vi "Display Results.vi"(8 "error in (no error)":errorcluster, 11 "Results in":refnum<class "Results.lvclass">) -> (0 "error out":errorcluster, 3 "Results out":refnum<class "Results.lvclass">)   [LabVIEW 2016, in "Result Actor.lvlib" / "Results.lvclass"]
uses:
  <userlib>/Common Components/Results/Results.lvclass
  <userlib>/Common Components/Results/Results.lvclass/Results.ctl
  <userlib>/Common Components/Results/Read Device Names Used.vi
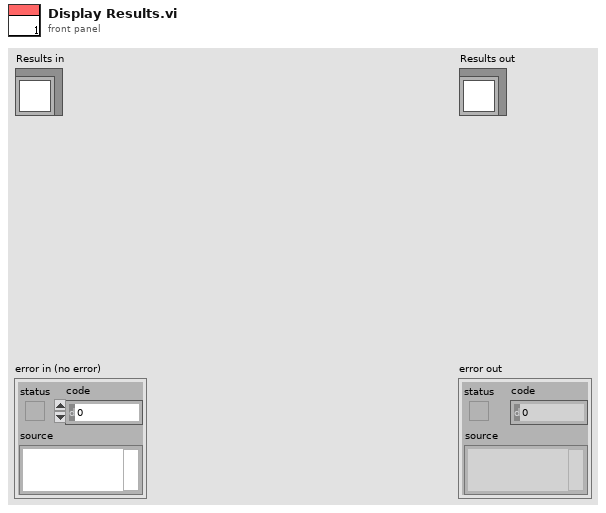
[diagram p1: front panel]
types:
  T1 = typedef "Result Actor.lvlib/Results.lvclass/UI References.ctl" = cluster{"Stop Button":refnum<vi>, "Waveform Graph":refnum<vi>, "Result Name":refnum<vi>, "Pass?":refnum<vi>}
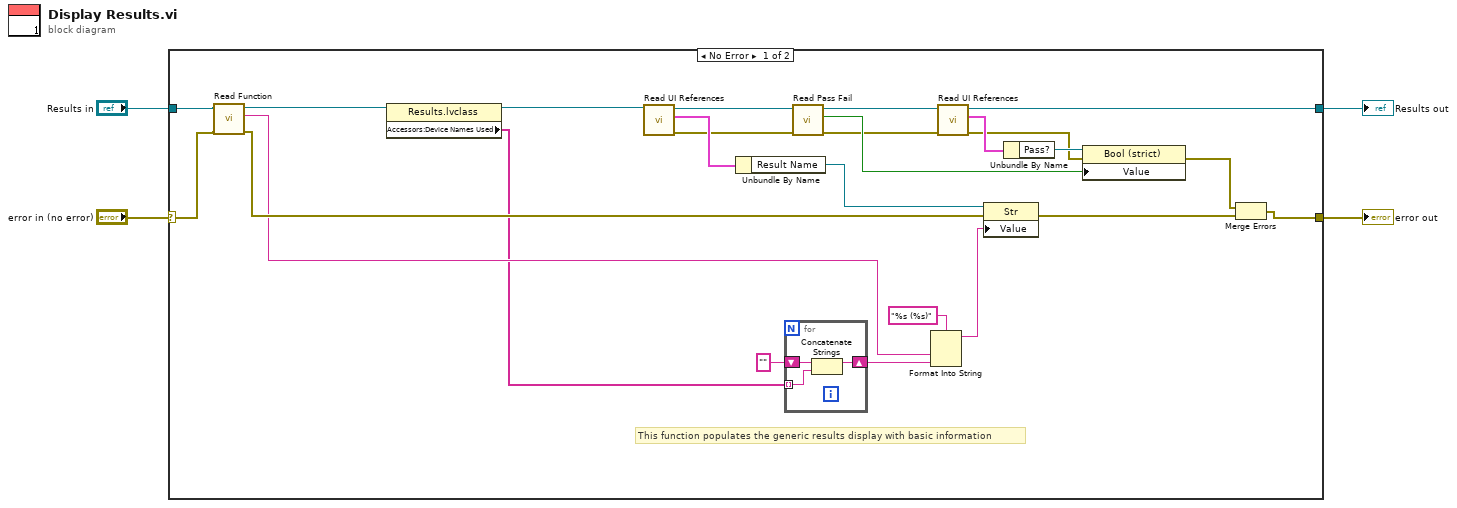
[diagram p0: block diagram]
diagram:
  n1 = case shown="No Error" "error in (no error)" {
    selector: "error in (no error)" -> [w10 w34]
    tunnel: [w25 w33] -> w2
    tunnel: "Results in" -> [w11 w33]
    tunnel: [w14 w34] -> w1
    frame No Error {
      # "This function populates the generic results display with basic information"
      n2 = call <userlib>:"Read Function.vi"("error in (no error)"=w10, "Results in"=w11) -> ("error out"=w9:errorcluster, "Function"=w8:string, "Results out"=w7:refnum<class "Results.lvclass">)  [unwired: 7 in]
      n3 = property class="Results.lvclass"(reference=w7) -> (reference out=w6:refnum<class "Results.lvclass">, "Accessors:Device Names Used"=w5:string[])  [unwired: 1 in, 1 out]
      n4 = call <userlib>:"Read UI References.vi"("Results in"=w6) -> ("error out"=w17:errorcluster, "UI References"=w29:T1, "Results out"=w24:refnum<class "Results.lvclass">)  [unwired: 8 in]
      n5 = Unbundle By Name(w29) -> ("Result Name"=w28:refnum<vi>)
      n6 = for {
        tunnel: w5 -> [w32] mode=indexing
        shift-right: [w31] -> w19
        shift-left: "" -> [w30]
        n7 = Concatenate Strings(w30, w32) -> (w31:string)
      }
      n8 = call <userlib>:"Read Pass Fail.vi"("error in (no error)"=w17, "Results in"=w24) -> ("error out"=w16:errorcluster, "Pass Fail"=w22:bool, "Results out"=w23:refnum<class "Results.lvclass">)  [unwired: 7 in]
      n9 = Format Into String(format string="%s (%s)" ("string"), w8, w19) -> (resulting string=w18:string)  [unwired: 2 in, 1 out]
      n10 = call <userlib>:"Read UI References.vi"("error in (no error)"=w16, "Results in"=w23) -> ("error out"=w15:errorcluster, "UI References"=w26:T1, "Results out"=w25:refnum<class "Results.lvclass">)  [unwired: 7 in]
      n11 = property class="Str"(reference=w28, error in=w9, "Value"=w18) -> (error out=w12:errorcluster)  [unwired: 1 out]
      n12 = Unbundle By Name(w26) -> ("Pass?"=w27:refnum<vi>)
      n13 = property class="Bool (strict)"(reference=w27, error in=w15, "Value"=w22) -> (error out=w13:errorcluster)  [unwired: 1 out]
      n14 = Merge Errors(w13, w12) -> (w14:errorcluster)
    }
    frame Error {
    }
  }
  "error out" <- w1
  "Results out" <- w2
